vi "Move to prepare stack.vi"(8 "error in (no error)":errorcluster, 11 "Tomo in":refnum<class "Tomo.lvclass">) -> (0 "error out":errorcluster, 3 "Tomo out":refnum<class "Tomo.lvclass">)   [LabVIEW 2012, in "Tomo.lvclass"]
uses:
  Tomo.lvclass
  <vilib>/Distrio/Murmex/GenericMessage/GenericMessage.lvclass
  <vilib>/Distrio/Murmex/StartMessage/StartMessage.lvclass
  <vilib>/Distrio/Murmex/Message/Message.lvclass
  <vilib>/Distrio/Murmex/Murmex/Murmex.lvclass
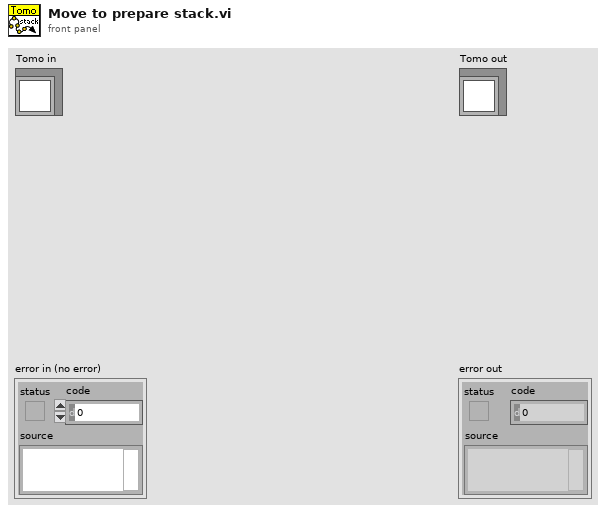
[diagram p1: front panel]
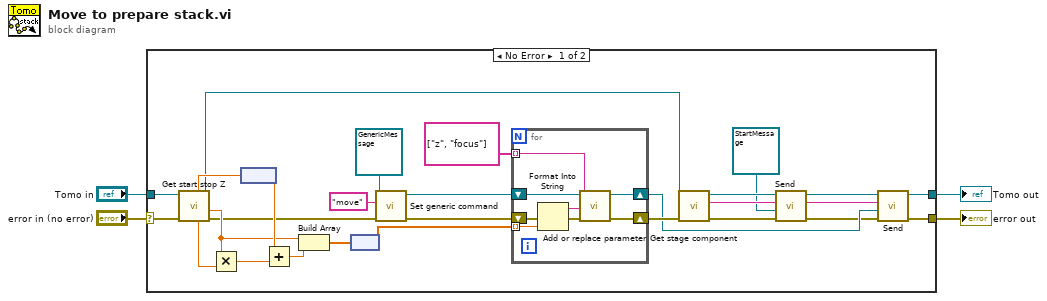
[diagram p0: block diagram]
diagram:
  n1 = case shown="No Error" "error in (no error)" {
    selector: "error in (no error)" -> [w30 w41]
    tunnel: [w8 w41] -> w3
    tunnel: [w7 w40] -> w1
    tunnel: "Tomo in" -> [w31 w40]
    frame No Error {
      n2 = call-dynamic "Get start stop Z.vi"("error in (no error)"=w30, "Tomo in"=w31) -> ("error out"=w9:errorcluster, "Z start"=w25:dbl[unit], "Tomo out"=w6:refnum<class "Tomo.lvclass">, "Focus slope"=w29:dbl, "Focus intercept"=w28:dbl)  [unwired: 4 in, 1 out]
      n3 = Multiply(x=w25, y=w29) -> (x*y=w27:dbl[unit])
      n4 = node(w28) -> (w26:dbl[unit])
      n5 = Add(x=w26, y=w27) -> (x+y=w24:dbl[unit])
      n6 = Build Array(w25, w24) -> (w23:dbl[unit][])
      n7 = node(w23) -> (w5:dbl[])
      n8 = call <vilib>:"Set generic command.vi"("error in (no error)"=w9, "generic command"="move" ("command string"), "GenericMessage in"=refnum<class "GenericMessage.lvclass"> refnum ("Murmex.lvlib:GenericMessage")) -> ("error out"=w20:errorcluster, "GenericMessage out"=w19:refnum<class "GenericMessage.lvclass">)  [unwired: 7 in]
      n9 = for {
        shift-right: [w33] -> w17
        shift-left: w20 -> [w39]
        shift-right: [w34] -> w16
        shift-left: w19 -> [w38]
        tunnel: string[] ["z", "focus"] -> [w36] mode=indexing
        tunnel: w5 -> [w35] mode=indexing
        n10 = Format Into String(error in=w39, w35) -> (resulting string=w32:string, error out=w37:errorcluster)  [unwired: 2 in]
        n11 = call <vilib>:"Add or replace parameter.vi"("error in (no error)"=w37, "value"=w32, "name"=w36, "Message in"=w38) -> ("error out"=w33:errorcluster, "Message out"=w34:refnum<class "GenericMessage.lvclass">)  [unwired: 6 in]
      }
      n12 = call-dynamic "Get stage component.vi"("error in (no error)"=w17, "Tomo in"=w6) -> ("error out"=w15:errorcluster, "stage component"=w11:string, "Tomo out"=w13:refnum<class "Tomo.lvclass">)  [unwired: 7 in]
      n13 = call <vilib>:"Send.vi"("error in (no error)"=w15, "Message"=refnum<class "StartMessage.lvclass"> refnum ("Distrio Murmex 1.1:StartMessage"), "recipient"=w11, "Murmex in"=w13) -> ("error out"=w14:errorcluster, "Murmex out"=w12:refnum<class "Tomo.lvclass">)  [unwired: 6 in]
      n14 = call <vilib>:"Send.vi"("error in (no error)"=w14, "Message"=w16, "recipient"=w11, "Murmex in"=w12) -> ("error out"=w8:errorcluster, "Murmex out"=w7:refnum<class "Tomo.lvclass">)  [unwired: 6 in]
    }
    frame Error {
    }
  }
  "error out" <- w3
  "Tomo out" <- w1
